vi "DriverStationGetCommands.vi"() -> ()   [LabVIEW 2020]
doc: "This VI receives instructions from the driver and manipulator controls, but only in certain robot modes. Specifically, these instructions are received while the robot is either \"running autonomously\" or in Super Test Mode. In all other robot modes, no instructions are received via the driver station. Instead they are output by the Autonomous Sequencer or completely disabled."
uses:
  GlobalAutonomous.vi
  GlobalDriverStationData.vi
  GlobalDriverStationCommands.vi
  GRNF_Joystick.vi
panel:
  in  "Buttons":bool[](array[boolean])=[FALSE, FALSE, FALSE, FALSE, FALSE, FALSE, FALSE, FALSE, FALSE, FALSE]
  in  "Right Trigger":dbl(slide) min=0.0 max=1.0 scale=0.0..1.0
  in  "Left Trigger":dbl(slide) min=0.0 max=1.0 step=0.1 scale=0.0..1.0
  in  "Right Joystick X":dbl(slide) scale=-1.0..1.0
  in  "Enable Joystick Control Override":bool
  in  "Joystick Left X":dbl(slide) scale=-1.0..1.0
  in  "Joystick Left Y":dbl(slide) scale=1.0..-1.0
  in  "Joystick Right Y":dbl(slide) scale=1.0..-1.0
  # "Left Thumbstick"
  # "Right Thumbstick"
  # "Driver A"
  # "Driver B"
  # "Driver X"
  # "Driver Y"
  # "Driver Left Bumper"
  # "Driver Right Bumper"
  # "Driver View"
  # "Driver Menu"
  # "Driver Left Joystick Button"
  # "Driver Right Joystick Button"
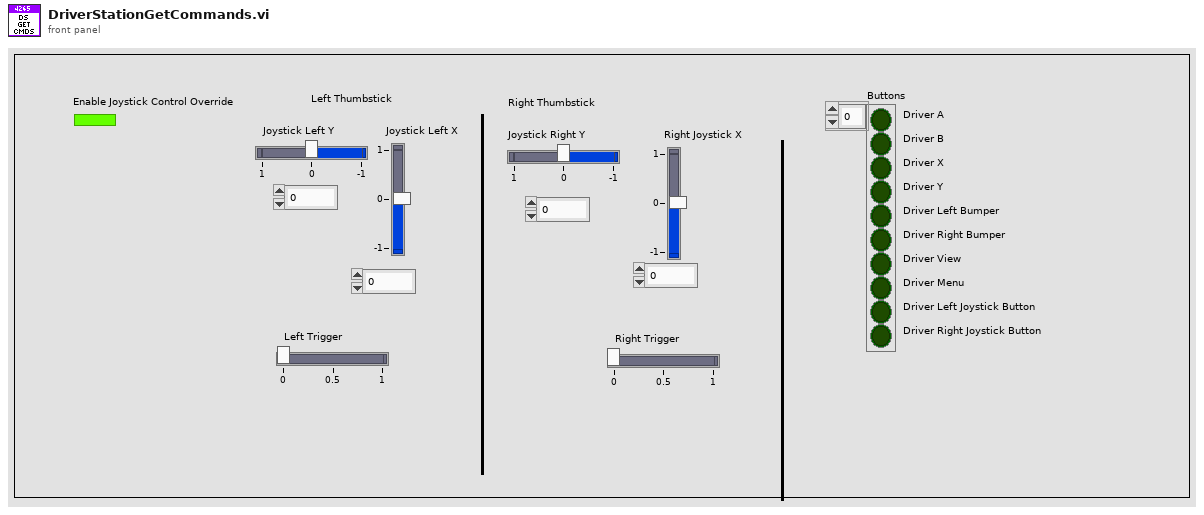
[diagram p1: front panel]
types:
  T1 = typedef "WPI_JoystickDevRef.ctl" = cluster{"Device":T2}
  T2 = typedef "WPI_JoystickDeviceEnum.ctl" = enum16{"USB 0", "USB 1", "USB 2", "USB 3", "USB 4", "USB 5"}
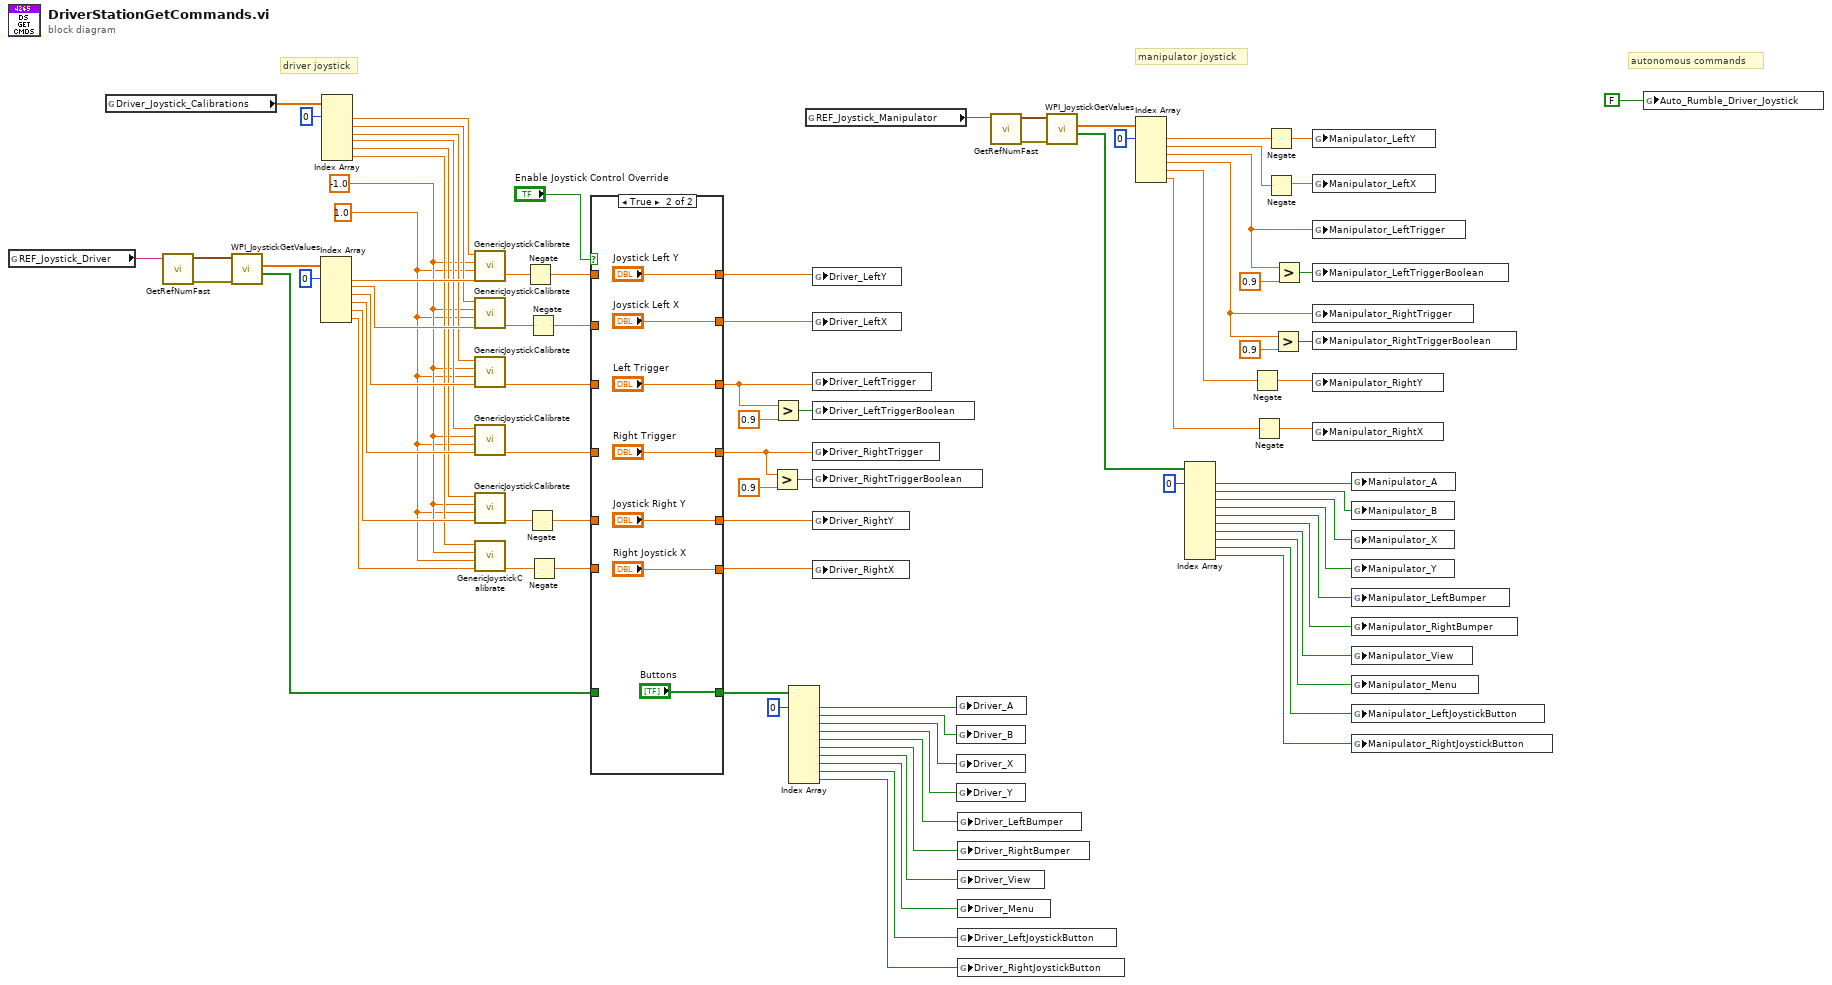
[diagram p0: block diagram]
diagram:
  w53 = 1.0
  w54 = -1.0
  # "manipulator joystick"
  # "autonomous commands"
  # "driver joystick"
  n1 = global read "GlobalDriverStationCommands.vi" "REF_Joystick_Driver"() -> (w2:string)
  n2 = global read "GlobalDriverStationData.vi" "Driver_Joystick_Calibrations"() -> (w71:dbl[])
  n3 = call-poly "GetRefNumFast.vi"("RefNum Name"=w2) -> ("Error"=w73:errorcluster, "Device Reference"=w74:T1)  [unwired: 5 in]
  n4 = call <vilib>:"WPI_JoystickGetValues.vi"("error in (no error)"=w73, "JoystickDevRef"=w74) -> ("Buttons"=w35:bool[], "Axes"=w87:dbl[])  [unwired: 5 in, 3 out]
  n5 = Index Array(array=w87, index #1=0 ("index")) -> (element #1=w66:dbl, element #2=w65:dbl, element #3=w61:dbl, element #4=w62:dbl, element #5=w63:dbl, element #6=w64:dbl)  [unwired: 5 in]
  n6 = Index Array(array=w71, index #1=0 ("index")) -> (element #1=w55:dbl, element #2=w56:dbl, element #3=w57:dbl, element #4=w58:dbl, element #5=w59:dbl, element #6=w60:dbl)  [unwired: 5 in]
  n7 = call "GenericJoystickCalibrate.vi"("Raw Joystick Value"=w66, "Maximum"=w53, "Minimum"=w54, "Deadband"=w55) -> ("Scaled Joystick Value"=w70:dbl)  [unwired: 3 in]
  n8 = call "GenericJoystickCalibrate.vi"("Raw Joystick Value"=w65, "Maximum"=w53, "Minimum"=w54, "Deadband"=w56) -> ("Scaled Joystick Value"=w69:dbl)  [unwired: 3 in]
  n9 = call "GenericJoystickCalibrate.vi"("Raw Joystick Value"=w61, "Maximum"=w53, "Minimum"=w54, "Deadband"=w57) -> ("Scaled Joystick Value"=w47:dbl)  [unwired: 3 in]
  n10 = call "GenericJoystickCalibrate.vi"("Raw Joystick Value"=w62, "Maximum"=w53, "Minimum"=w54, "Deadband"=w58) -> ("Scaled Joystick Value"=w41:dbl)  [unwired: 3 in]
  n11 = call "GenericJoystickCalibrate.vi"("Raw Joystick Value"=w63, "Maximum"=w53, "Minimum"=w54, "Deadband"=w59) -> ("Scaled Joystick Value"=w68:dbl)  [unwired: 3 in]
  n12 = call "GenericJoystickCalibrate.vi"("Raw Joystick Value"=w64, "Maximum"=w53, "Minimum"=w54, "Deadband"=w60) -> ("Scaled Joystick Value"=w67:dbl)  [unwired: 3 in]
  n13 = Negate(x=w70) -> (-x=w50:dbl)
  n14 = Negate(x=w68) -> (-x=w38:dbl)
  n15 = Negate(x=w69) -> (-x=w49:dbl)
  n16 = Negate(x=w67) -> (-x=w37:dbl)
  n17 = case shown="True" "Enable Joystick Control Override" {
    tunnel: w47 -> [w92 _]
    tunnel: [w94 "Joystick Left Y"] -> w51
    tunnel: w50 -> [w94 _]
    tunnel: [w93 "Joystick Left X"] -> w48
    tunnel: w49 -> [w93 _]
    tunnel: [w92 "Left Trigger"] -> w42
    tunnel: w41 -> [w91 _]
    tunnel: [w91 "Right Trigger"] -> w40
    tunnel: [w90 "Joystick Right Y"] -> w39
    tunnel: w38 -> [w90 _]
    tunnel: [w89 "Right Joystick X"] -> w36
    tunnel: w37 -> [w89 _]
    tunnel: w35 -> [w88 _]
    tunnel: [w88 "Buttons"] -> w34
    frame False {
    }
    frame True {
    }
  }
  n18 = Greater?(x=w40, y=0.9) -> (0:w44:bool)
  n19 = Greater?(x=w42, y=0.9) -> (0:w43:bool)
  n20 = Index Array(array=w34, index #1=0 ("index")) -> (element #1=w84:bool, element #2=w83:bool, element #3=w82:bool, element #4=w81:bool, element #5=w80:bool, element #6=w79:bool, element #7=w78:bool, element #8=w77:bool, element #9=w76:bool, element #10=w75:bool)  [unwired: 9 in]
  n21 = global read "GlobalDriverStationCommands.vi" "REF_Joystick_Manipulator"() -> (w1:string)
  n22 = global write "GlobalDriverStationCommands.vi" "Driver_LeftY"(w51) -> ()
  n23 = global write "GlobalDriverStationCommands.vi" "Driver_LeftX"(w48) -> ()
  n24 = global write "GlobalDriverStationCommands.vi" "Driver_LeftTrigger"(w42) -> ()
  n25 = global write "GlobalDriverStationCommands.vi" "Driver_LeftTriggerBoolean"(w43) -> ()
  n26 = global write "GlobalDriverStationCommands.vi" "Driver_RightTrigger"(w40) -> ()
  n27 = global write "GlobalDriverStationCommands.vi" "Driver_RightTriggerBoolean"(w44) -> ()
  n28 = global write "GlobalDriverStationCommands.vi" "Driver_RightY"(w39) -> ()
  n29 = global write "GlobalDriverStationCommands.vi" "Driver_RightX"(w36) -> ()
  n30 = global write "GlobalDriverStationCommands.vi" "Driver_A"(w84) -> ()
  n31 = global write "GlobalDriverStationCommands.vi" "Driver_B"(w83) -> ()
  n32 = global write "GlobalDriverStationCommands.vi" "Driver_X"(w82) -> ()
  n33 = global write "GlobalDriverStationCommands.vi" "Driver_Y"(w81) -> ()
  n34 = global write "GlobalDriverStationCommands.vi" "Driver_LeftBumper"(w80) -> ()
  n35 = global write "GlobalDriverStationCommands.vi" "Driver_RightBumper"(w79) -> ()
  n36 = global write "GlobalDriverStationCommands.vi" "Driver_View"(w78) -> ()
  n37 = global write "GlobalDriverStationCommands.vi" "Driver_Menu"(w77) -> ()
  n38 = global write "GlobalDriverStationCommands.vi" "Driver_LeftJoystickButton"(w76) -> ()
  n39 = global write "GlobalDriverStationCommands.vi" "Driver_RightJoystickButton"(w75) -> ()
  n40 = call-poly "GetRefNumFast.vi"("RefNum Name"=w1) -> ("Error"=w18:errorcluster, "Device Reference"=w19:T1)  [unwired: 5 in]
  n41 = call <vilib>:"WPI_JoystickGetValues.vi"("error in (no error)"=w18, "JoystickDevRef"=w19) -> ("Buttons"=w4:bool[], "Axes"=w32:dbl[])  [unwired: 5 in, 3 out]
  n42 = Index Array(array=w32, index #1=0 ("index")) -> (element #1=w17:dbl, element #2=w16:dbl, element #3=w3:dbl, element #4=w13:dbl, element #5=w14:dbl, element #6=w15:dbl)  [unwired: 5 in]
  n43 = Index Array(array=w4, index #1=0 ("index")) -> (element #1=w29:bool, element #2=w28:bool, element #3=w27:bool, element #4=w26:bool, element #5=w25:bool, element #6=w24:bool, element #7=w23:bool, element #8=w22:bool, element #9=w21:bool, element #10=w20:bool)  [unwired: 9 in]
  n44 = Negate(x=w14) -> (-x=w6:dbl)
  n45 = Negate(x=w15) -> (-x=w5:dbl)
  n46 = Negate(x=w17) -> (-x=w12:dbl)
  n47 = Negate(x=w16) -> (-x=w11:dbl)
  n48 = Greater?(x=w13, y=0.9) -> (0:w8:bool)
  n49 = Greater?(x=w3, y=0.9) -> (0:w7:bool)
  n50 = global write "GlobalDriverStationCommands.vi" "Manipulator_LeftY"(w12) -> ()
  n51 = global write "GlobalDriverStationCommands.vi" "Manipulator_LeftX"(w11) -> ()
  n52 = global write "GlobalDriverStationCommands.vi" "Manipulator_LeftTrigger"(w3) -> ()
  n53 = global write "GlobalDriverStationCommands.vi" "Manipulator_LeftTriggerBoolean"(w7) -> ()
  n54 = global write "GlobalDriverStationCommands.vi" "Manipulator_RightTrigger"(w13) -> ()
  n55 = global write "GlobalDriverStationCommands.vi" "Manipulator_RightTriggerBoolean"(w8) -> ()
  n56 = global write "GlobalDriverStationCommands.vi" "Manipulator_RightY"(w6) -> ()
  n57 = global write "GlobalDriverStationCommands.vi" "Manipulator_RightX"(w5) -> ()
  n58 = global write "GlobalDriverStationCommands.vi" "Manipulator_A"(w29) -> ()
  n59 = global write "GlobalDriverStationCommands.vi" "Manipulator_B"(w28) -> ()
  n60 = global write "GlobalDriverStationCommands.vi" "Manipulator_X"(w27) -> ()
  n61 = global write "GlobalDriverStationCommands.vi" "Manipulator_Y"(w26) -> ()
  n62 = global write "GlobalDriverStationCommands.vi" "Manipulator_LeftBumper"(w25) -> ()
  n63 = global write "GlobalDriverStationCommands.vi" "Manipulator_RightBumper"(w24) -> ()
  n64 = global write "GlobalDriverStationCommands.vi" "Manipulator_View"(w23) -> ()
  n65 = global write "GlobalDriverStationCommands.vi" "Manipulator_Menu"(w22) -> ()
  n66 = global write "GlobalDriverStationCommands.vi" "Manipulator_LeftJoystickButton"(w21) -> ()
  n67 = global write "GlobalDriverStationCommands.vi" "Manipulator_RightJoystickButton"(w20) -> ()
  n68 = global write "GlobalAutonomous.vi" "Auto_Rumble_Driver_Joystick"(FALSE ("Auto_Force_To_Low_Gear")) -> ()
